vi "Update Display.vi"(6 "Priority Message? (F)":bool, 8 "error in":errorcluster, 11 "Message string":string) -> (0 "error out":errorcluster)   [LabVIEW 2015]
uses:
  Message Queue/Message Queue.lvlib
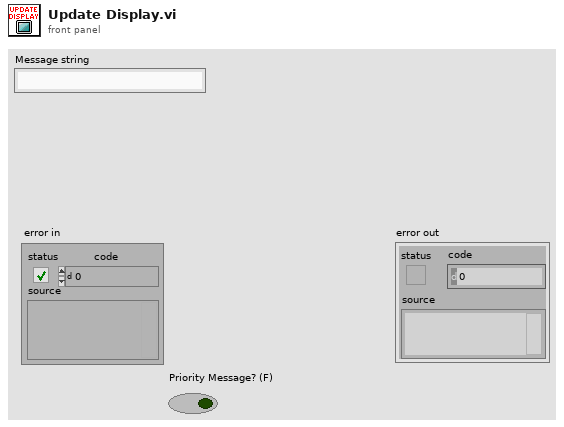
[diagram p1: front panel]
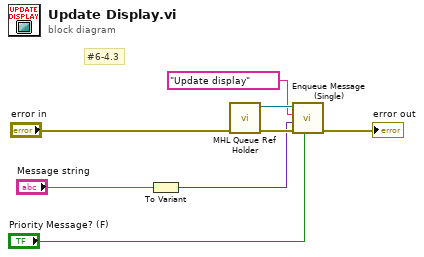
[diagram p0: block diagram]
diagram:
  # "#6-4.3"
  n1 = To Variant(anything="Message string") -> (Variant=w1:variant)
  n2 = call "MHL Queue Ref Holder.vi"("error in"="error in") -> ("error out"=w4:errorcluster, "Input Message Queue"=w6:refnum<queue>)  [unwired: 9 in]
  n3 = call "Enqueue Message (Single).vi"("Priority Message? (F)"="Priority Message? (F)", "error in (no error)"=w4, "Message Data"=w1, "Message"="Update display", "Message Queue"=w6) -> ("error out"=→"error out":errorcluster)  [unwired: 5 in, 1 out]
